vi "run_starting_set_v02.vi"(8 "error in":errorcluster, 9 "data in":T1={"daq_ao 1"="Dev1/ao0", "daq_ai 1"="Dev1/ai0", "experiment day folder"=path "D:/DATA/8-27-15 save func testing/test.lvm", "Multiclamp init error"=0, "Multiclamp Handle Out"=0, "sampling rate (Hz)"=10000, "trial name"=""}, 11 "controls array in":refnum<vi>[](array[refnum])) -> (0 "error out":errorcluster, 1 "data out":T1={"daq_ao 1"="Dev1/ao0", "daq_ai 1"="Dev1/ai0", "experiment day folder"=path "D:/DATA/8-27-15 save func testing/test.lvm", "Multiclamp init error"=0, "Multiclamp Handle Out"=0, "sampling rate (Hz)"=10000, "trial name"=""}, 3 "control array out":refnum<vi>[](array[refnum]))   [LabVIEW 2015]
uses:
  get_data_from_control_tfarray.vi
  get_data_from_control_double.vi
  Controls/Data.ctl
panel:
  out "starting TF set":T2
  # "RUN STARTING SET AUTO WC"
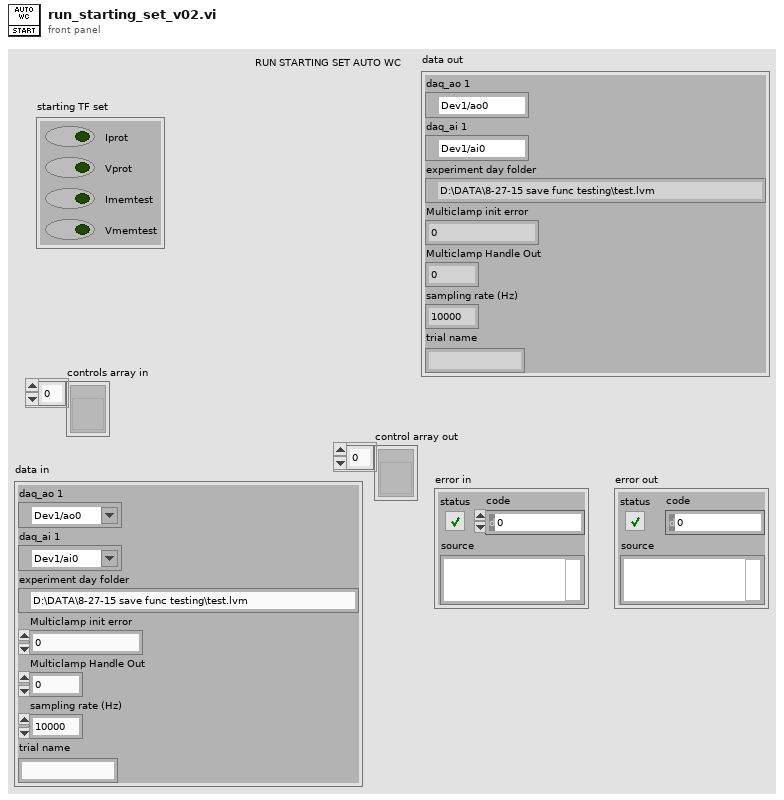
[diagram p1: front panel]
types:
  T1 = typedef "Data.ctl" = cluster{"daq_ao 1":tag, "daq_ai 1":tag, "experiment day folder":path, "Multiclamp init error":i32, "Multiclamp Handle Out":u32, "sampling rate (Hz)":i32, "trial name":string}
  T2 = cluster{" Iprot":bool, " Vprot":bool, " Imemtest":bool, " Vmemtest":bool}
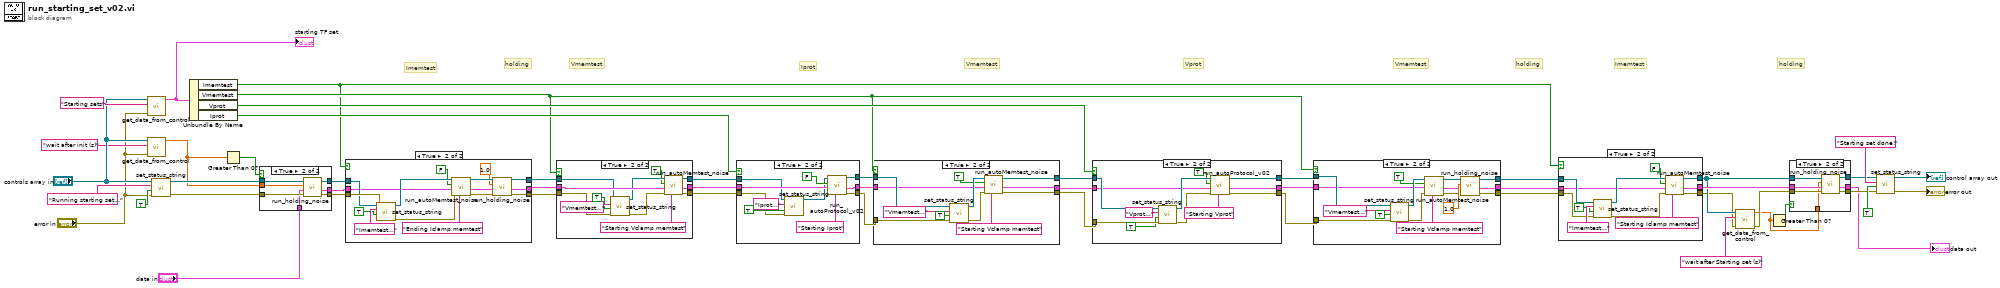
[diagram p0: block diagram]
diagram:
  # "Imemtest"
  # "Vmemtest"
  # "Vmemtest"
  # "holding"
  # "Vmemtest"
  # "holding"
  # "holding"
  # "Imemtest"
  # "Vprot"
  # "Iprot"
  n1 = call-poly "get_data_from_control.vi"("error in"="error in", "control label"="Starting sets", "controls array"="controls array in") -> ("TF set out"=w51:T2)  [unwired: 7 in, 1 out]
  "starting TF set" <- w51
  n2 = call-poly "get_data_from_control.vi"("error in"="error in", "control label"="wait after init (s)", "controls array"="controls array in") -> ("double out"=w4:dbl)  [unwired: 7 in, 1 out]
  n3 = call "set_status_string.vi"("error in"="error in", "new line?"=TRUE, "status string in"="Running starting set...", "controls array"="controls array in") -> ("error out"=w18:errorcluster, "controls array out"=w19:refnum<vi>[])  [unwired: 6 in]
  n4 = Unbundle By Name(w51) -> ("Imemtest"=w29:bool, "Vmemtest"=w30:bool, "Vprot"=w37:bool, "Iprot"=w50:bool)
  n5 = Greater Than 0?(x=w4) -> (x > 0?=w3:bool)
  n6 = case shown="True" w3 {
    tunnel: w19 -> [w54 w61]
    tunnel: w18 -> [w53 w60]
    tunnel: [w53 w59] -> w17
    tunnel: [w54 w58] -> w16
    tunnel: "data in" -> [w52 w57]
    tunnel: [w52 w56] -> w14
    tunnel: w4 -> [_ w55]
    frame False {
    }
    frame True {
      n7 = call "run_holding_noise.vi"("error in"=w60, "data in"=w57, "holding time (s)"=w55, "controls array in"=w61) -> ("error out"=w59:errorcluster, "data out"=w56:T1, "controls array out"=w58:refnum<vi>[])  [unwired: 4 in, 1 out]
    }
  }
  n8 = case shown="True" w29 {
    tunnel: [w64 w67] -> w8
    tunnel: [w62 w65] -> w10
    tunnel: [w63 w66] -> w9
    tunnel: w17 -> [w62 w74]
    tunnel: w16 -> [w64 w73]
    tunnel: w14 -> [w63 w72]
    frame False {
    }
    frame True {
      n9 = call "set_status_string.vi"("error in"=w74, "new line?"=TRUE, "status string in"="Imemtest...", "controls array"=w73) -> ("error out"=w76:errorcluster, "controls array out"=w79:refnum<vi>[])  [unwired: 6 in]
      n10 = call "run_autoMemtest_noise.vi"("control label"="Ending Iclamp memtest", "error in"=w76, "data in"=w72, "clamp switch (T=v, F=i)"=FALSE, "controls array"=w79) -> ("error out"=w70:errorcluster, "data out"=w69:T1, "controls out"=w71:refnum<vi>[])  [unwired: 2 in, 2 out]
      n11 = call "run_holding_noise.vi"("error in"=w70, "data in"=w69, "holding time (s)"=1.0, "controls array in"=w71) -> ("error out"=w65:errorcluster, "data out"=w66:T1, "controls array out"=w67:refnum<vi>[])  [unwired: 4 in, 1 out]
    }
  }
  n12 = case shown="True" w30 {
    tunnel: w8 -> [w83 w94]
    tunnel: w10 -> [w81 w90]
    tunnel: w9 -> [w82 w95]
    tunnel: [w83 w88] -> w46
    tunnel: [w82 w87] -> w45
    tunnel: [w81 w86] -> w44
    frame False {
    }
    frame True {
      n13 = call "set_status_string.vi"("error in"=w90, "new line?"=TRUE, "status string in"="Vmemtest...", "controls array"=w94) -> ("error out"=w89:errorcluster, "controls array out"=w93:refnum<vi>[])  [unwired: 6 in]
      n14 = call "run_autoMemtest_noise.vi"("control label"="Starting Vclamp memtest", "error in"=w89, "data in"=w95, "clamp switch (T=v, F=i)"=TRUE, "controls array"=w93) -> ("error out"=w86:errorcluster, "data out"=w87:T1, "controls out"=w88:refnum<vi>[])  [unwired: 2 in, 2 out]
    }
  }
  n15 = case shown="True" w50 {
    tunnel: w46 -> [w98 w103]
    tunnel: w45 -> [w96 w106]
    tunnel: w44 -> [w97 w107]
    tunnel: [w98 w101] -> w40
    tunnel: [w97 w100] -> w39
    tunnel: [w96 w99] -> w38
    frame False {
    }
    frame True {
      n16 = call "set_status_string.vi"("error in"=w107, "new line?"=TRUE, "status string in"="Iprot...", "controls array"=w103) -> ("controls array out"=w102:refnum<vi>[])  [unwired: 6 in, 1 out]
      n17 = call "run_autoProtocol_v02.vi"("control label"="Starting Iprot", "data in"=w106, "clamp switch (T=v, F=i)"=FALSE, "controls array"=w102) -> ("error out"=w100:errorcluster, "data out"=w99:T1, "controls array out"=w101:refnum<vi>[])  [unwired: 5 in]
    }
  }
  n18 = case shown="True" w30 {
    tunnel: w40 -> [w112 w124]
    tunnel: w39 -> [w110 w122]
    tunnel: w38 -> [w111 w119]
    tunnel: [w112 w115] -> w36
    tunnel: [w110 w114] -> w35
    tunnel: [w111 w113] -> w34
    frame False {
    }
    frame True {
      n19 = call "set_status_string.vi"("error in"=w122, "new line?"=TRUE, "status string in"="Vmemtest...", "controls array"=w124) -> ("error out"=w121:errorcluster, "controls array out"=w123:refnum<vi>[])  [unwired: 6 in]
      n20 = call "run_autoMemtest_noise.vi"("control label"="Starting Vclamp memtest", "error in"=w121, "data in"=w119, "clamp switch (T=v, F=i)"=TRUE, "controls array"=w123) -> ("error out"=w114:errorcluster, "data out"=w113:T1, "controls out"=w115:refnum<vi>[])  [unwired: 2 in, 2 out]
    }
  }
  n21 = case shown="True" w37 {
    tunnel: w36 -> [w127 w139]
    tunnel: w35 -> [w125 w138]
    tunnel: w34 -> [w126 w132]
    tunnel: [w127 w130] -> w33
    tunnel: [w126 w129] -> w32
    tunnel: [w125 w128] -> w31
    frame False {
    }
    frame True {
      n22 = call "set_status_string.vi"("error in"=w138, "new line?"=TRUE, "status string in"="Vprot...", "controls array"=w139) -> ("error out"=w135:errorcluster, "controls array out"=w136:refnum<vi>[])  [unwired: 6 in]
      n23 = call "run_autoProtocol_v02.vi"("control label"="Starting Vprot", "error in"=w135, "data in"=w132, "clamp switch (T=v, F=i)"=TRUE, "controls array"=w136) -> ("error out"=w128:errorcluster, "data out"=w129:T1, "controls array out"=w130:refnum<vi>[])  [unwired: 4 in]
    }
  }
  n24 = case shown="True" w30 {
    tunnel: w33 -> [w142 w158]
    tunnel: w31 -> [w140 w156]
    tunnel: w32 -> [w141 w153]
    tunnel: [w142 w148] -> w7
    tunnel: [w140 w143] -> w5
    tunnel: [w141 w144] -> w6
    frame False {
    }
    frame True {
      n25 = call "set_status_string.vi"("error in"=w156, "new line?"=TRUE, "status string in"="Vmemtest...", "controls array"=w158) -> ("error out"=w155:errorcluster, "controls array out"=w157:refnum<vi>[])  [unwired: 6 in]
      n26 = call "run_autoMemtest_noise.vi"("control label"="Starting Vclamp memtest", "error in"=w155, "data in"=w153, "clamp switch (T=v, F=i)"=TRUE, "controls array"=w157) -> ("error out"=w146:errorcluster, "data out"=w145:T1, "controls out"=w149:refnum<vi>[])  [unwired: 2 in, 2 out]
      n27 = call "run_holding_noise.vi"("error in"=w146, "data in"=w145, "holding time (s)"=1.0, "controls array in"=w149) -> ("error out"=w143:errorcluster, "data out"=w144:T1, "controls array out"=w148:refnum<vi>[])  [unwired: 4 in, 1 out]
    }
  }
  n28 = case shown="True" w29 {
    tunnel: w7 -> [w161 w173]
    tunnel: w5 -> [w160 w165]
    tunnel: [w161 w169] -> w23
    tunnel: [w160 w168] -> w21
    tunnel: [w159 w167] -> w28
    tunnel: w6 -> [w159 w162]
    frame False {
    }
    frame True {
      n29 = call "set_status_string.vi"("error in"=w165, "new line?"=TRUE, "status string in"="Imemtest...", "controls array"=w173) -> ("error out"=w164:errorcluster, "controls array out"=w171:refnum<vi>[])  [unwired: 6 in]
      n30 = call "run_autoMemtest_noise.vi"("control label"="Starting Iclamp memtest", "error in"=w164, "data in"=w162, "clamp switch (T=v, F=i)"=FALSE, "controls array"=w171) -> ("error out"=w168:errorcluster, "data out"=w167:T1, "controls out"=w169:refnum<vi>[])  [unwired: 2 in, 2 out]
    }
  }
  n31 = call-poly "get_data_from_control.vi"("error in"=w21, "control label"="wait after Starting set (s)", "controls array"=w23) -> ("error out"=w20:errorcluster, "double out"=w1:dbl)  [unwired: 7 in]
  n32 = Greater Than 0?(x=w1) -> (x > 0?=w2:bool)
  n33 = case shown="True" w2 {
    tunnel: w28 -> [w175 w183]
    tunnel: [w176 w182] -> w27
    tunnel: [w174 w181] -> w26
    tunnel: [w175 w180] -> w25
    tunnel: w23 -> [w176 w179]
    tunnel: w20 -> [w174 w178]
    tunnel: w1 -> [_ w177]
    frame False {
    }
    frame True {
      n34 = call "run_holding_noise.vi"("error in"=w178, "data in"=w183, "holding time (s)"=w177, "controls array in"=w179) -> ("error out"=w181:errorcluster, "data out"=w180:T1, "controls array out"=w182:refnum<vi>[])  [unwired: 4 in, 1 out]
    }
  }
  "data out" <- w25
  n35 = call "set_status_string.vi"("error in"=w26, "new line?"=TRUE, "status string in"="Starting set done!", "controls array"=w27) -> ("error out"=→"error out":errorcluster, "controls array out"=→"control array out":refnum<vi>[])  [unwired: 6 in]
